vi "MsgUnpack.vi"(8 "error in (no error)":errorcluster, 11 "connection":refnum<k5>) -> (0 "error out":errorcluster, 1 "msg_id":u16, 2 "msg_type":T1, 3 "connection out":refnum<k5>, 4 "msg_len":u16)   [LabVIEW 2014]
uses:
  MsgType.ctl
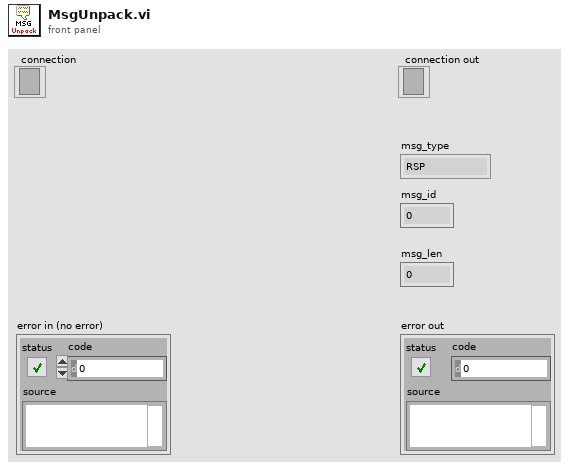
[diagram p1: front panel]
types:
  T1 = typedef "MsgType.ctl" = enum8{"RSP", "REGISTER", "LOGIN", "SAVE_PROF", "LOAD_PROF", "GET_TOKEN", "PING", "ACTIVATE", "DEACTIVATE", "REFRESH", "UNDEFINED0", "UNDEFINED1", "TWEET", "EMAIL", "NOTIFY", "BRIDGE", "UNDEFINED2", "UNDEFINED3", "UNDEFINED4", "UNDEFINED5", "HW"}
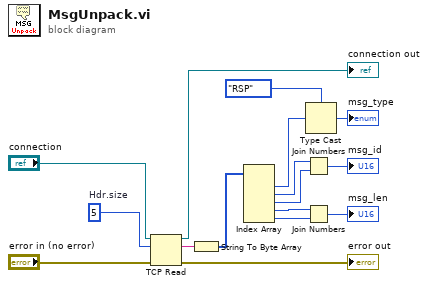
[diagram p0: block diagram]
diagram:
  w16 = 5  # Hdr.size
  n1 = TCP Read(connection ID="connection", bytes to read=w16, error in (no error)="error in (no error)") -> (connection ID out=→"connection out":refnum<k5>, data out=w15:string, error out=→"error out":errorcluster)  [unwired: 2 in]
  n2 = String To Byte Array(string=w15) -> (unsigned byte array=w14:u8[])
  n3 = Index Array(array=w14) -> (element #1=w2:u8, element #2=w9:u8, element #3=w8:u8, element #4=w5:u8, element #5=w4:u8)  [unwired: 5 in]
  n4 = Join Numbers(hi=w9, lo=w8) -> ((hi.lo)=→"msg_id":u16)
  n5 = Join Numbers(hi=w5, lo=w4) -> ((hi.lo)=→"msg_len":u16)
  n6 = Type Cast(type=MsgType."RSP", x=w2) -> (*(type *) &x=→"msg_type":T1)
